vi "test Scheduled Loopback Value Overflow.vi"(8 "error in":errorcluster, 11 "TestCase in":refnum<class "Single Board Loopback.lvclass">) -> (0 "error out":errorcluster, 3 "TestCase out":refnum<class "Single Board Loopback.lvclass">)   [LabVIEW 2020, in "Single Board Loopback.lvclass"]
uses:
  Single Board Loopback.lvclass
  <vilib>/addons/_JKI Toolkits/VI Tester/TestCase.llb/TestCase.lvclass
  <vilib>/NI VeriStand/Execution/Workspace/NI_VS Workspace ExecutionAPI.lvlib
  <vilib>/NI/VeriStand Custom Device Testing Tools/VeriStandTestUtilities/VeriStandTestUtilities.lvlib
  <vilib>/numeric/Random Number (Range) U64.vi
  <vilib>/NI VeriStand/Execution/Workspace/NI VeriStand - Set Multiple Channel Values.vi
  C:/Program Files (x86)/National Instruments/LabVIEW 2020/vi.lib/addons/_JKI Toolkits/VI Tester/TestCase.llb/TestCase.lvclass
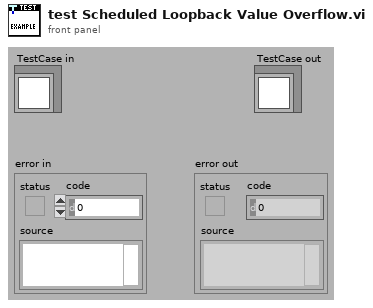
[diagram p1: front panel]
types:
  T1 = typedef "NI_VS Workspace ExecutionAPI.lvlib/WorkspaceAPI.ctl" = refnum<k24>
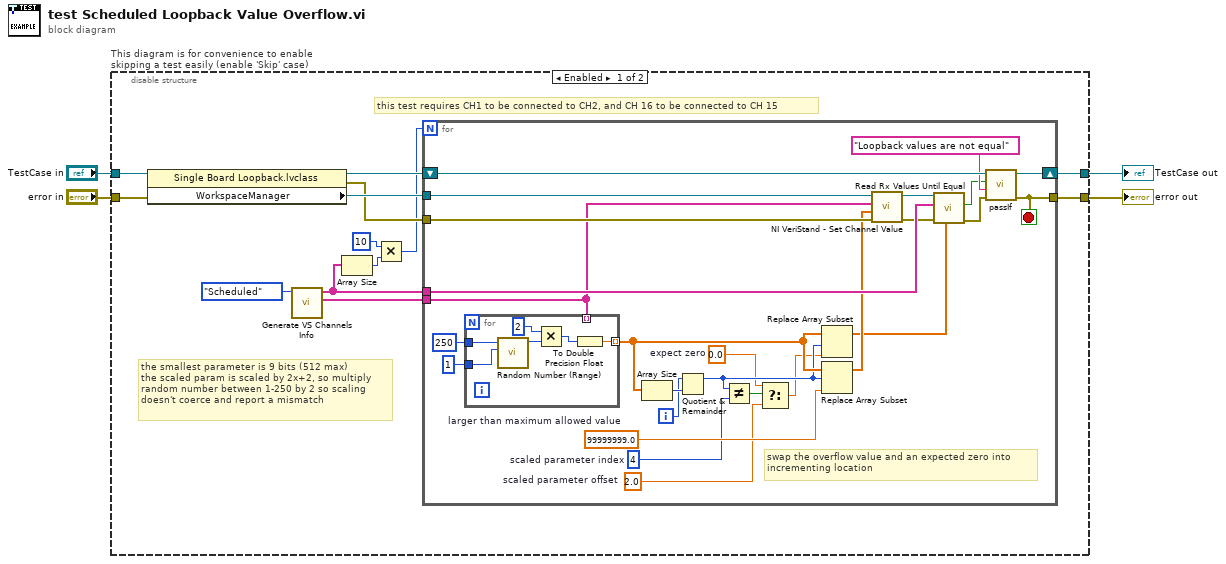
[diagram p0: block diagram]
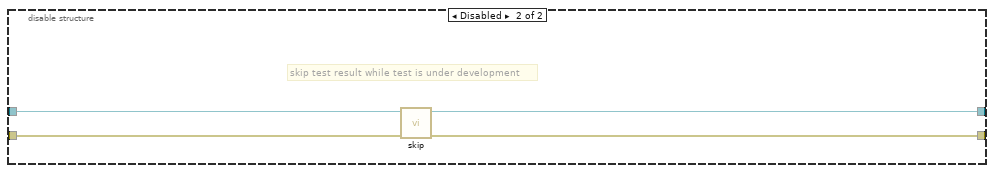
[diagram p2: hidden frame]
diagram:
  n1 = disable-structure "This diagram is for convenience to enable skipping a test easily (enable 'Skip' case)" shown="Enabled" {
    disable-tunnel: "TestCase in" -> [w14 w53]
    disable-tunnel: [w12 w51] -> w1
    disable-tunnel: [w11 w52] -> w3
    disable-tunnel: "error in" -> [w13 w50]
    frame Enabled {
      # "the smallest parameter is 9 bits (512 max)\nthe scaled param is scaled by 2x+2, so multiply \nrandom number between 1-250 by 2 so scaling\ndoesn't coerce and report a mismatch"
      # "this test requires CH1 to be connected to CH2, and CH 16 to be connected to CH 15"
      n2 = property class="Single Board Loopback.lvclass"(reference=w14, error in=w13) -> (reference out=w15:refnum<class "Single Board Loopback.lvclass">, error out=w16:errorcluster, "WorkspaceManager"=w17:T1)
      n3 = call "Generate VS Channels Info.vi"("Transfer Type"=enum16{"Acyclic", "Scheduled"}."Scheduled") -> ("Tx Channels Array"=w10:string[], "Rx Channels Array"=w9:string[])  [unwired: 6 in, 3 out]
      n4 = Array Size(array=w9) -> (size(s)=w8:i32)
      n5 = Multiply(x=10, y=w8) -> (x*y=w6:i32)
      n6 = for {
        N: w6 -> [_]
        tunnel: w9 -> [w36]
        tunnel: w17 -> [w30]
        tunnel: w16 -> [w35]
        tunnel: w10 -> [w29]
        shift-right: [w42] -> w12
        shift-left: w15 -> [w43]
        tunnel: [w41] -> w11
        i -> [w24]
        stop <- w41 stop-if-true
        w19 = 2.0  # scaled parameter offset
        w22 = 4  # scaled parameter index
        w20 = 0.0  # expect zero
        w37 = 99999999.0  # larger than maximum allowed value
        # "swap the overflow value and an expected zero into \nincrementing location"
        n7 = for {
          tunnel: [w48] -> w25 mode=indexing
          tunnel: u64 250 ("upper bound (100)") -> [w47]
          tunnel: u64 1 ("upper bound (100)") -> [w46]
          tunnel: w29 -> [_] mode=indexing
          n8 = call-poly <vilib>:"Random Number (Range).vi"("lower bound (0)"=w46, "upper bound (100)"=w47) -> ("number"=w49:u64)  [unwired: 9 in]
          n9 = Multiply(x=u64 2, y=w49) -> (x*y=w45:u64)
          n10 = To Double Precision Float(number=w45) -> (double precision float=w48:dbl)
        }
        n11 = Array Size(array=w25) -> (size(s)=w26:i32)
        n12 = Quotient & Remainder(x=w24, y=w26) -> (x-y*floor(x/y)=w23:i32)  [unwired: 1 out]
        n13 = Not Equal?(x=w23, y=w22) -> (x != y?=w21:bool)
        n14 = Select(t=w20, s=w21, f=w19) -> (s? t:f=w18:dbl)
        n15 = Replace Array Subset(array=w25, new element=w18, index=w23) -> (w27:dbl[])
        n16 = Replace Array Subset(array=w25, new element=w37, index=w23) -> (w28:dbl[])
        n17 = call-poly <vilib>:"NI VeriStand - Set Channel Value.vi"("error in (no error)"=w35, "Values"=w28, "Channels"=w29, "WorkspaceManager in"=w30) -> ("error out"=w34:errorcluster, "WorkspaceManager out"=w31:T1)  [unwired: 6 in]
        n18 = call <vilib>:"Read Rx Values Until Equal.vi"("expected values"=w27, "error in"=w34, "Rx aliases"=w36, "workspace manager in"=w31) -> ("error out"=w33:errorcluster, "values equal expected"=w32:bool)  [unwired: 5 in, 1 out]
        n19 = call-dynamic "passIf.vi"("error in (no error)"=w33, "message (\"\")"="Loopback values are not equal" ("message (\"\")"), "pass"=w32, "TestCase in"=w43) -> ("error out"=w41:errorcluster, "TestCase out"=w42:refnum<class "Single Board Loopback.lvclass">)  [unwired: 6 in]
      }
    }
    frame Disabled {
      # "skip test result while test is under development"
      n20 = call <vilib>:"skip.vi"("error in (no error)"=w50, "TestCase in"=w53) -> ("error out"=w52:errorcluster, "TestCase out"=w51:refnum<class "Single Board Loopback.lvclass">)  [unwired: 8 in]
    }
  }
  "error out" <- w3
  "TestCase out" <- w1
